vi "Update Script.vi"   [LabVIEW 2016, in "Apple script.lvlib"]
doc: "Updates the script periodically. Put this in the disable vi."
uses:
  <vilib>/Rock Robotics/Network Tables/NT Write Number.vi
  Apple script.lvlib
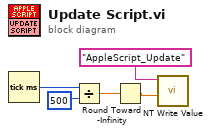
[diagram p0: block diagram]
diagram:
  n1 = Tick Count (ms)() -> (millisecond timer value=w5:u32)
  n2 = Divide(x=w5, y=u32 500) -> (x/y=w3:dbl)
  n3 = Round Toward -Infinity(1:w3) -> (0:w1:dbl)
  n4 = call-poly <vilib>:"NT Write Value.vi"("Numeric"=w1, "Name"="AppleScript_Update") -> ()  [unwired: 9 in, 1 out]
